vi "Laser 1 Operations L3 compute next state.vi"() -> ()   [LabVIEW 2017]
uses:
  Global Variables/General Globals.vi
  Type Defs/Ls1 Operations.ctl
panel:
  out "Next State":T1
  in  "Shutter Changed ?":bool
  in  "Wavelength Changed ?":bool
  in  "Previous State":T1
  in  "Current State":T1
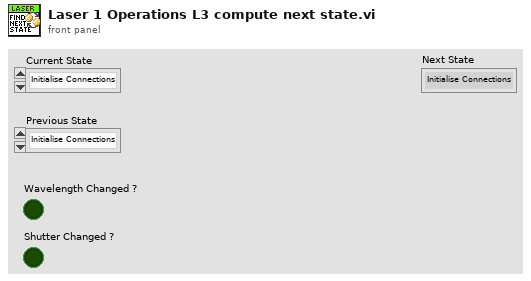
[diagram p1: front panel]
types:
  T1 = typedef "Ls1 Operations.ctl" = enum16{"Initialise Connections", "Initialise system", "Check Status", "Open/Close Shutter", "Start/Stop Pump Peak Hold", "Set wavelength", "Close"}
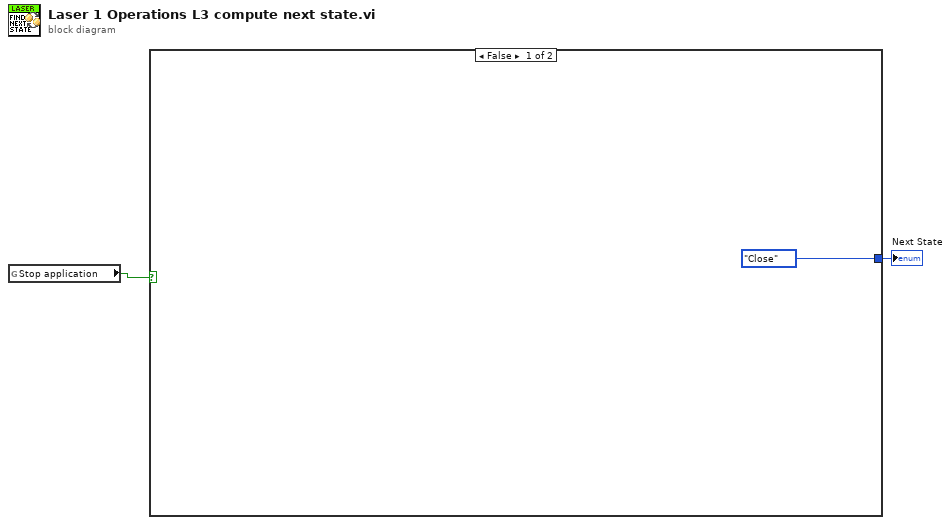
[diagram p0: block diagram]
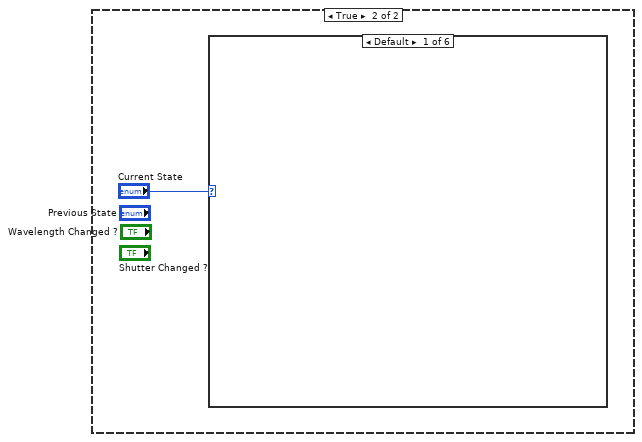
[diagram p2: hidden frame]
diagram:
  n1 = global read "General Globals.vi" "Stop application"() -> (w2:bool)
  n2 = case shown="False" w2 {
    tunnel: [Ls1_Operations."Close" ("Current State 2") _] -> w1
    frame False {
    }
    frame True {
      n3 = case shown="Default" "Current State" {
        frame Default {
        }
        frame "Check Status" {
        }
        frame "Open/Close Shutter" {
        }
        frame "Start/Stop Pump Peak Hold" {
        }
        frame "Set wavelength" {
        }
        frame "Close" {
        }
      }
    }
  }
  "Next State" <- w1
